vi "Write UUID.vi"(10 "UUID":string, 11 "UniqueName in":refnum<class "UniqueName.lvclass">) -> (3 "UniqueName out":refnum<class "UniqueName.lvclass">)   [LabVIEW 2014, in "UniqueName.lvlib" / "UniqueName.lvclass"]
uses:
  UniqueName.lvclass
  UniqueName.lvclass/UniqueName.ctl
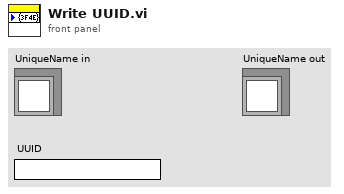
[diagram p1: front panel]
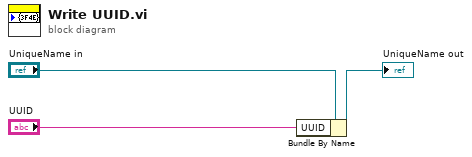
[diagram p0: block diagram]
diagram:
  n1 = Bundle By Name(cluster="UniqueName in", "UUID"="UUID") -> (→"UniqueName out":refnum<class "UniqueName.lvclass">)
